vi "HistoPlotter.vi"(0 "Filtered Histogram":T1, 1 "Add in":bool, 3 "Reset in":bool, 5 "Outside":cluster{"total":i32, "below":i32, "above":i32}, 9 "Array":dbl[](array[numeric]), 12 "min":dbl, 13 "max":dbl, 14 "Voltage Bins":i32) -> (4 "Histogram Graph":T1, 6 "# outside":cluster{"total":i32, "below":i32, "above":i32})   [LabVIEW 2017]
uses:
  <vilib>/Analysis/NI_AALPro.lvlib
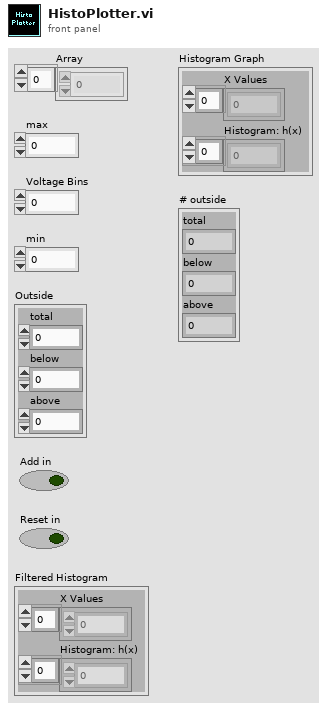
[diagram p1: front panel]
types:
  T1 = cluster{"X Values":dbl[], "Histogram: h(x)":i32[]}
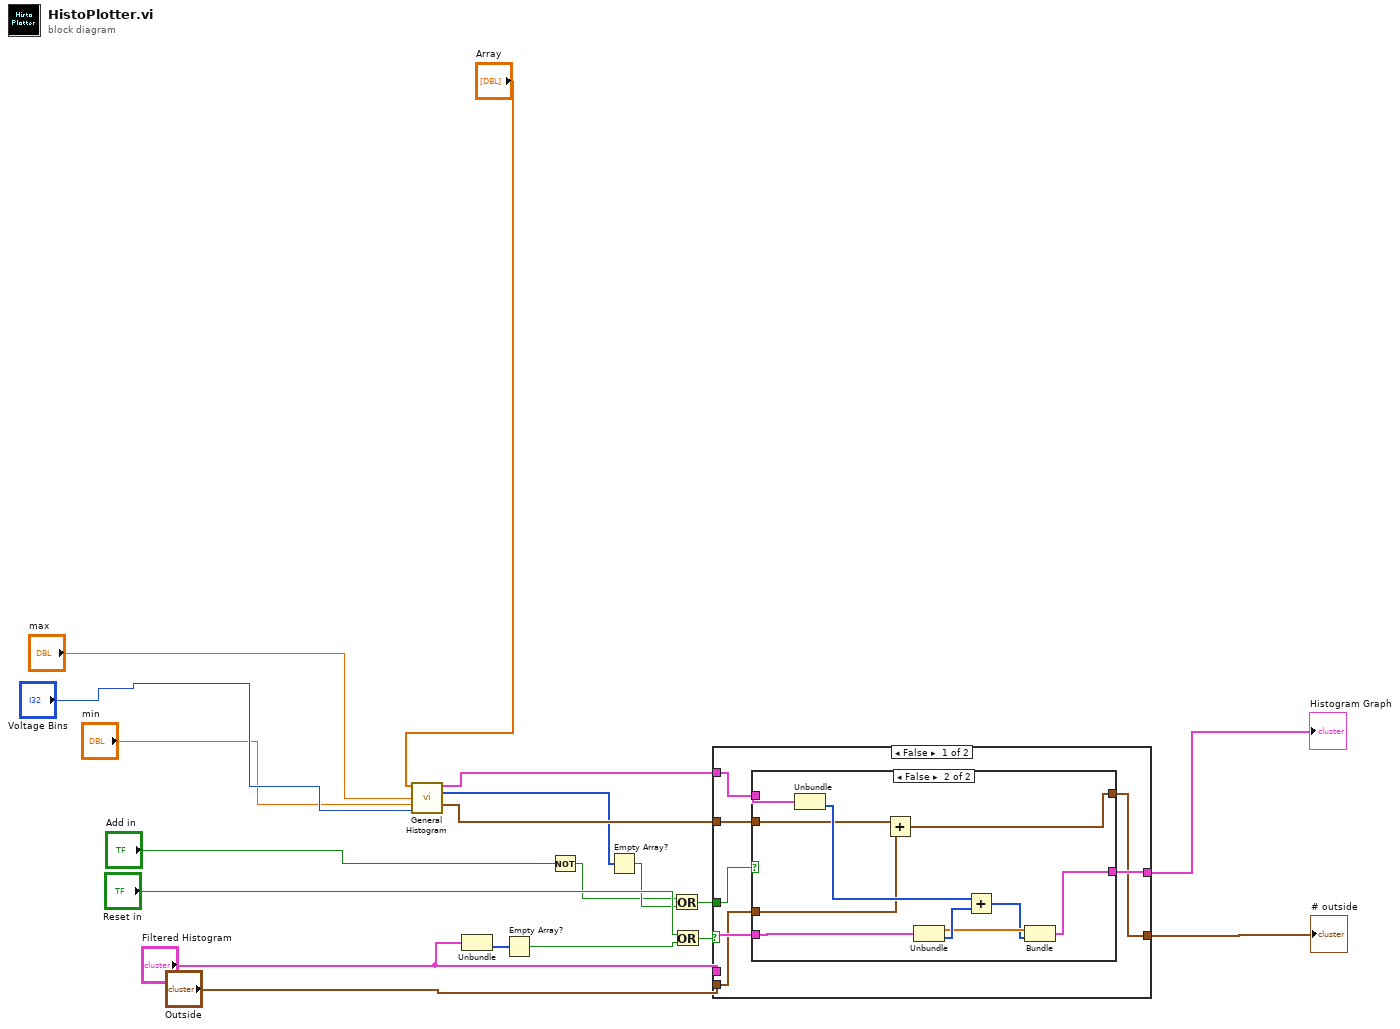
[diagram p0: block diagram]
diagram:
  n1 = call <vilib>:"General Histogram.vi"("X"="Array", "max"="max", "min"="min", "# bins"="Voltage Bins") -> ("Histogram Graph"=w10:T1, "Histogram"=w9:i32[], "# outside"=w11:cluster{"total":i32, "below":i32, "above":i32})  [unwired: 7 in, 2 out]
  n2 = Unbundle("Filtered Histogram") -> ("Histogram: h(x)"=w6:i32[])  [unwired: 1 out]
  n3 = Empty Array?(array=w6) -> (empty?=w5:bool)
  n4 = Not(x="Add in") -> (.not. x?=w1:bool)
  n5 = Empty Array?(array=w9) -> (empty?=w2:bool)
  n6 = Or(x=w1, y=w2) -> (x .or. y?=w3:bool)
  n7 = Or(x="Reset in", y=w5) -> (x .or. y?=w4:bool)
  n8 = case shown="False" w4 {
    tunnel: [w26 w40] -> w12
    tunnel: w3 -> [w25 _]
    tunnel: [w24 w39] -> w15
    tunnel: w10 -> [w23 w40]
    tunnel: w11 -> [w22 w39]
    tunnel: "Filtered Histogram" -> [w21 _]
    tunnel: "Outside" -> [w20 _]
    frame False {
      n9 = case shown="False" w25 {
        tunnel: [w28 w35] -> w26
        tunnel: [w27 w34] -> w24
        tunnel: w23 -> [_ w33]
        tunnel: w22 -> [_ w31]
        tunnel: w21 -> [w28 w30]
        tunnel: w20 -> [w27 w29]
        frame True {
        }
        frame False {
          n10 = Unbundle(w33) -> ("Histogram: h(x)"=w32:i32[])  [unwired: 1 out]
          n11 = Add(x=w31, y=w29) -> (x+y=w34:cluster{"total":i32, "below":i32, "above":i32})
          n12 = Unbundle(w30) -> ("X Values"=w37:dbl[], "Histogram: h(x)"=w38:i32[])
          n13 = Add(x=w32, y=w38) -> (x+y=w36:i32[])
          n14 = Bundle("X Values"=w37, w36) -> (w35:cluster{"X Values":dbl[], i32[]})  [unwired: 1 in]
        }
      }
    }
    frame True {
    }
  }
  "# outside" <- w15
  "Histogram Graph" <- w12
